vi "ReadGpio.vi"(8 "error in (no error)":errorcluster, 11 "FpgaInterface in":refnum<class "FpgaInterface.lvclass">) -> (0 "error out":errorcluster, 1 "GPIO #2 out":u32, 2 "GPIO #1 out":u32, 3 "FpgaInterface out":refnum<class "FpgaInterface.lvclass">)   [LabVIEW 2017, in "FpgaInterface.lvclass"]
uses:
  FpgaInterface.lvclass
  FpgaInterface.lvclass/FpgaInterface.ctl
  <vilib>/Utility/error.llb/Error Cluster From Error Code.vi
  <vilib>/rvi/errors/niLvFpgaAdjustHostInterfaceError.vi
  <vilib>/rvi/interface/nirviReadWriteControl/nirviReadWriteControl.xnode
  NiFpgaLv.dll
  <vilib>/rvi/interface/Simulation/niFpgaSimulationCallBeginRW.vi
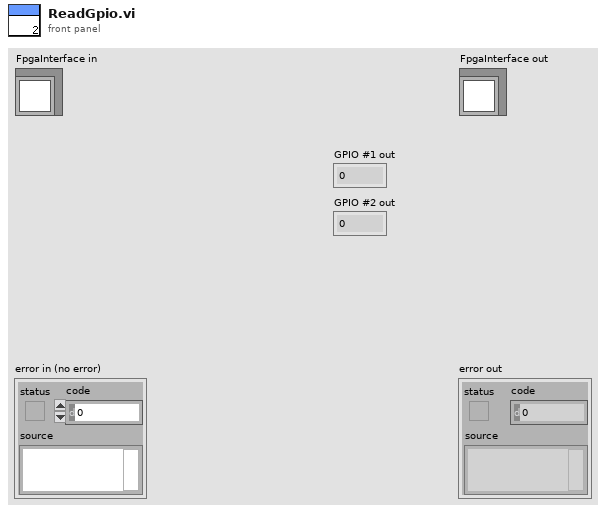
[diagram p1: front panel]
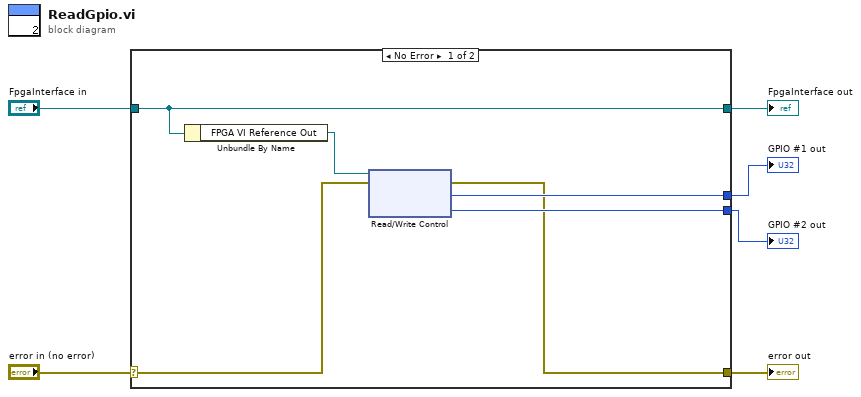
[diagram p0: block diagram]
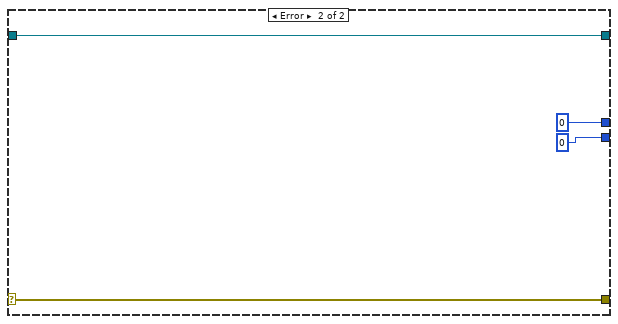
[diagram p2: hidden frame]
diagram:
  n1 = case shown="No Error" "error in (no error)" {
    selector: "error in (no error)" -> [w10 w16]
    tunnel: [w7 w16] -> w5
    tunnel: [w12 w15] -> w3
    tunnel: "FpgaInterface in" -> [w12 w15]
    tunnel: [w9 u32 0 ("GPIO #1 out")] -> w2
    tunnel: [w8 u32 0 ("GPIO #2 out")] -> w1
    frame No Error {
      n2 = Unbundle By Name(w12) -> ("FPGA VI Reference Out"=w11:refnum<k20>)
      n3 = xnode "Read/Write Control"("FPGA VI Reference In"=w11, "error in"=w10) -> ("error out"=w7:errorcluster, "GPIO #1 out"=w9:u32, "GPIO #2 out"=w8:u32)  [unwired: 1 out]
    }
    frame Error {
    }
  }
  "error out" <- w5
  "FpgaInterface out" <- w3
  "GPIO #1 out" <- w2
  "GPIO #2 out" <- w1
